vi "HandleDrive.vi"(10 "DriveInstruction":T1, 11 "Deadzone":dbl=0.15) -> (2 "DriveInstruction":T1, 3 "Enqueue?":bool)   [LabVIEW 2013]
doc: "Determines whether to enqueue a drive instruction. \nIf either joystick is outside the deadzone or half/straight drive is flipped, Enqueue? outputs true.\nIf the joysticks have just entered the deadzone, the motor outputs are set to 0 and Enqueue? outputs true.\nIf they are still in the deadzone (and previously were), Enqueue? outputs false."
uses:
  DriveData.ctl
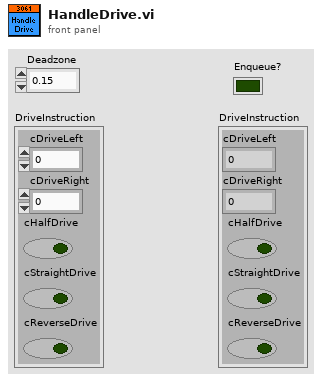
[diagram p1: front panel]
types:
  T1 = typedef "DriveData.ctl" = cluster{"cDriveLeft":dbl, "cDriveRight":dbl, "cHalfDrive":bool, "cStraightDrive":bool, "cReverseDrive":bool}
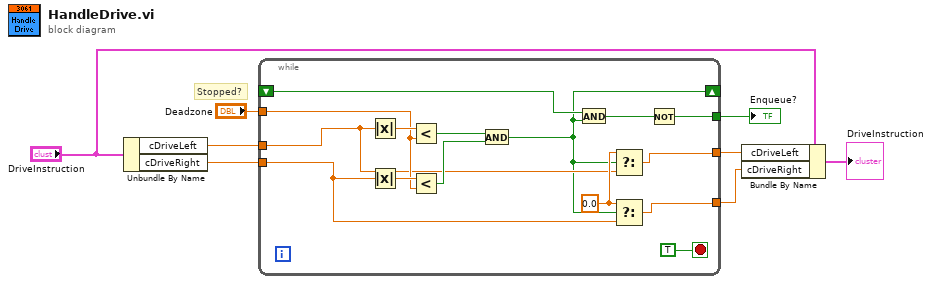
[diagram p0: block diagram]
diagram:
  # "Stopped?"
  n1 = Unbundle By Name("DriveInstruction") -> ("cDriveLeft"=w6:dbl, "cDriveRight"=w5:dbl)
  n2 = while {
    tunnel: w6 -> [w15]
    tunnel: "Deadzone" -> [w21]
    tunnel: [w20] -> w3
    tunnel: [w19] -> w2
    shift-right: [w9] -> _
    shift-left: _ -> [w14]
    tunnel: [w13] -> w7
    tunnel: w5 -> [w10]
    stop <- TRUE stop-if-true
    w16 = 0.0
    n3 = Absolute Value(x=w15) -> (abs(x)=w22:dbl)
    n4 = Absolute Value(x=w10) -> (abs(x)=w23:dbl)
    n5 = Less?(x=w22, y=w21) -> (x < y?=w18:bool)
    n6 = Less?(x=w23, y=w21) -> (x < y?=w17:bool)
    n7 = And(x=w18, y=w17) -> (x .and. y?=w9:bool)
    n8 = And(x=w14, y=w9) -> (x .and. y?=w12:bool)
    n9 = Select(t=w16, s=w9, f=w15) -> (s? t:f=w20:dbl)
    n10 = Select(t=w16, s=w9, f=w10) -> (s? t:f=w19:dbl)
    n11 = Not(x=w12) -> (.not. x?=w13:bool)
  }
  "Enqueue?" <- w7
  n12 = Bundle By Name(cluster="DriveInstruction", "cDriveLeft"=w3, "cDriveRight"=w2) -> (→"DriveInstruction":T1)
